vi "Get Joint Array.vi"(8 "error in":errorcluster, 10 "Tree Elements":T1[](array[typedef]), 11 "Scene In":refnum<vi>) -> (0 "error out":errorcluster, 2 "Joint Array":T4[](array[typedef]), 3 "Scene Out":refnum<vi>)   [LabVIEW 2017, in "NI_Robotics_3DKinematics.lvlib"]
uses:
  <vilib>/robotics/Kinematics/Plotting/NI_Robotics_3DKinematics.lvlib
  <vilib>/robotics/Kinematics/Plotting/Joint Control.ctl
  <vilib>/robotics/Kinematics/Plotting/Joint Type.ctl
  <vilib>/robotics/Kinematics/Plotting/Tree Element.ctl
  <vilib>/robotics/Kinematics/Plotting/Element Type.ctl
  <vilib>/picture/3D Picture Control/NI_3D Picture Control.lvlib
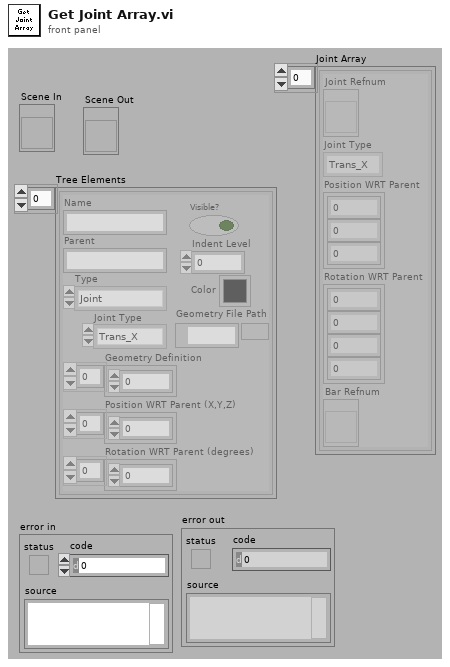
[diagram p1: front panel]
types:
  T1 = typedef "NI_Robotics_3DKinematics.lvlib/Tree Element.ctl" = cluster{"Name":string, "Parent":string, "Type":T2, "Visible?":bool, "Geometry Definition":dbl[], "Position WRT Parent (X,Y,Z)":dbl[], "Rotation WRT Parent (degrees)":dbl[], "Joint Type":T3, "Geometry File Path":path, "Indent Level":i32, "Color":u32}
  T2 = typedef "NI_Robotics_3DKinematics.lvlib/Element Type.ctl" = enum16{"Joint", "Box", "Cylinder", "Cone", "Sphere", "ASE File", "VRML File", "STL File", "Space"}
  T3 = typedef "NI_Robotics_3DKinematics.lvlib/Joint Type.ctl" = enum16{"Trans_X", "Trans_Y", "Trans_Z", "Rot_X", "Rot_Y", "Rot_Z", "None"}
  T4 = typedef "NI_Robotics_3DKinematics.lvlib/Joint Control.ctl" = cluster{"Joint Refnum":refnum<vi>, "Joint Type":T3, "Position WRT Parent":dbl[], "Rotation WRT Parent":dbl[], "Bar Refnum":refnum<vi>}
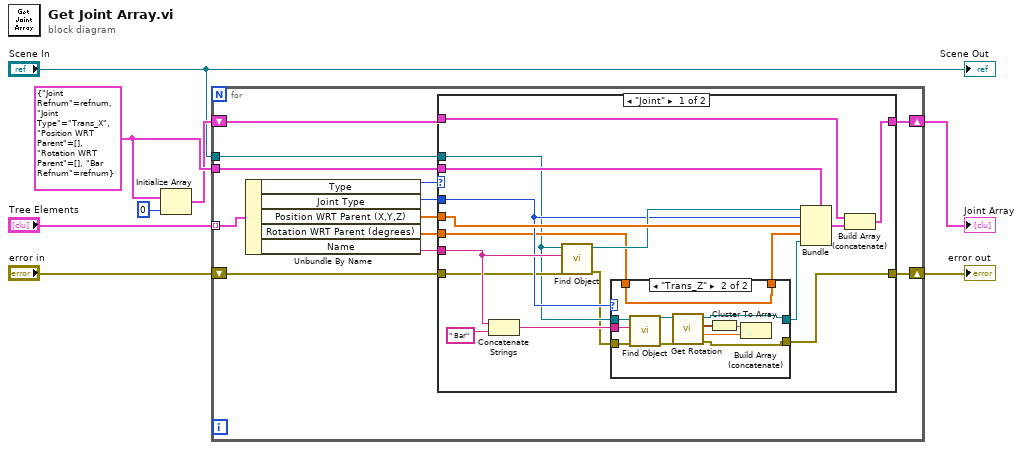
[diagram p0: block diagram]
diagram:
  w7 = T4 {"Joint Refnum"=refnum, "Joint Type"=enum."Trans_X", "Position WRT Parent"=[], "Rotation WRT Parent"=[], "Bar Refnum"=refnum} ("Joints")
  n1 = Initialize Array(w7, 0 ("dimension size")) -> (w6:T4[])
  n2 = for {
    tunnel: "Scene In" -> [w20]
    tunnel: "Tree Elements" -> [w19] mode=indexing
    shift-right: [w15] -> w8
    shift-left: w6 -> [w16]
    tunnel: w7 -> [w17]
    shift-right: [w14] -> w2
    shift-left: "error in" -> [w18]
    n3 = Unbundle By Name(w19) -> ("Type"=w12:T2, "Joint Type"=w11:T3, "Position WRT Parent (X,Y,Z)"=w10:dbl[], "Rotation WRT Parent (degrees)"=w9:dbl[], "Name"=w13:string)
    n4 = case shown="\"Joint\"" w12 {
      tunnel: w20 -> [w24 _]
      tunnel: w13 -> [w31 _]
      tunnel: w18 -> [w26 w53]
      tunnel: [w22 w53] -> w14
      tunnel: w11 -> [w29 _]
      tunnel: w17 -> [w37 _]
      tunnel: w16 -> [w35 w52]
      tunnel: [w34 w52] -> w15
      tunnel: w10 -> [w33 _]
      tunnel: w9 -> [w28 _]
      frame "Joint" {
        n5 = Concatenate Strings(w31, " Bar" ("string")) -> (w25:string)
        n6 = call <vilib>:"Find Object.vi"("error in (no error)"=w26, "Object Name"=w31, "Scene Refnum"=w24) -> ("error out"=w23:errorcluster, "Object Refnum"=w30:refnum<vi>)  [unwired: 7 out]
        n7 = case shown="\"Trans_Z\"" w29 {
          tunnel: w28 -> [w40 w41]
          tunnel: [w40 w41] -> w27
          tunnel: w25 -> [_ w48]
          tunnel: w24 -> [w38 w47]
          tunnel: w23 -> [w39 w45]
          tunnel: [w39 w43] -> w22
          tunnel: [w38 w42] -> w21
          frame Default {
          }
          frame "Trans_Z" {
            n8 = call <vilib>:"Find Object.vi"("error in (no error)"=w45, "Object Name"=w48, "Scene Refnum"=w47) -> ("error out"=w44:errorcluster, "Object Refnum"=w46:refnum<vi>)  [unwired: 7 out]
            n9 = call <vilib>:"Get Rotation.vi"("error in (no error)"=w44, "Scene Object"=w46) -> ("error out"=w43:errorcluster, "Angle"=w49:sgl, "Axis"=w51:cluster{"X":sgl, "Y":sgl, "Z":sgl}, "Scene Object"=w42:refnum<vi>)  [unwired: 6 in]
            n10 = Cluster To Array(cluster=w51) -> (array=w50:sgl[])
            n11 = Build Array (concatenate)(w50, w49) -> ()  [unwired: 1 out]
          }
        }
        n12 = Bundle(cluster=w37, "Joint Refnum"=w30, "Joint Type"=w29, "Position WRT Parent"=w33, "Rotation WRT Parent"=w27, "Bar Refnum"=w21) -> (w36:T4)
        n13 = Build Array (concatenate)(w35, w36) -> (w34:T4[])
      }
      frame Default {
      }
    }
  }
  "Joint Array" <- w8
  "error out" <- w2
  "Scene Out" <- "Scene In"
